vi "Auto Setup.vi"(4 "Sequence Context":T2) -> (0 "error out":errorcluster, 1 "Test Data":T1={"PASS/FAIL Flag"=TRUE, "Numeric Measurement"=0.0, "String Measurement"="", "Report Text"=""} {"Numeric Measurement" format="%.2f"})   [LabVIEW 2013]
uses:
  <vilib>/addons/TestStand/_TSLegacy.llb/LabVIEW Test - Sequence Context.ctl
  <vilib>/addons/TestStand/_TSLegacy.llb/LabVIEW Test - Test Data.ctl
panel:
  in  "Power Train Control Module":bool
  in  "Engine Control Module":bool=TRUE
  in  "Fuel Injection":bool
  in  "Ignition System":bool=TRUE
  in  "Charging System":bool
  in  "Accept":bool
  in  "Battery Voltage":dbl(knob)=11.72609352032594 scale=0.0..15.0 scale format="%.1f"
  # "Verify sequence algorithm by setting tests to Fail.\nForce test(s) to Fail by clicking the appropriate checkbox."
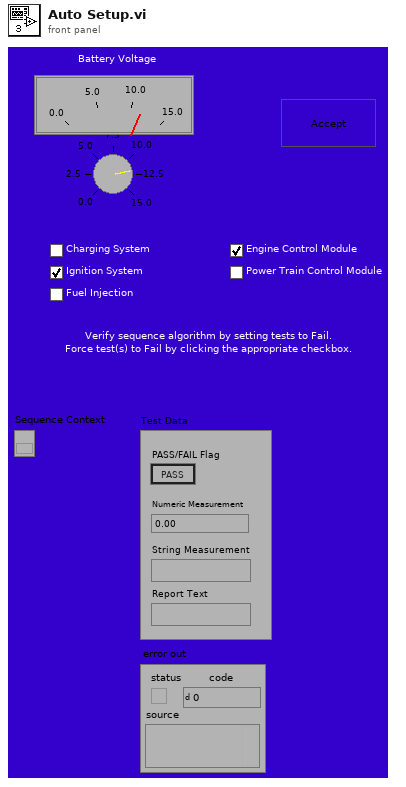
[diagram p1: front panel]
types:
  T1 = typedef "LabVIEW Test - Test Data.ctl" = cluster{"PASS/FAIL Flag":bool, "Numeric Measurement":dbl, "String Measurement":string, "Report Text":string}
  T2 = typedef "LabVIEW Test - Sequence Context.ctl" = refnum<k7>
  T3 = typedef "TestStand - Status Monitor.ctl" = cluster{"Sequence Context":refnum<k7>, "Execution":refnum<k7>, "Termination Monitor":refnum<k7>}
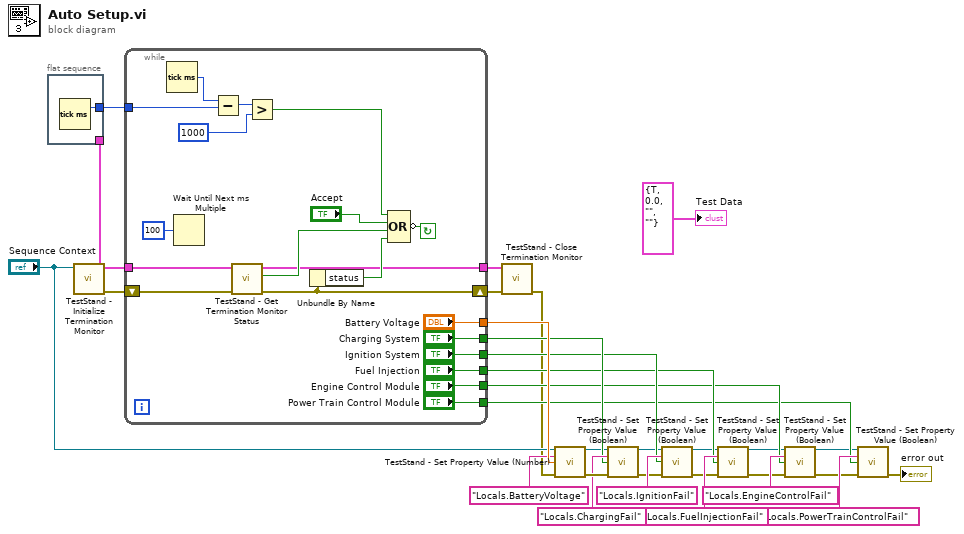
[diagram p0: block diagram]
diagram:
  n1 = flat-sequence {
    tunnel: [w32] -> w1
    tunnel: w2 -> [_]
    frame #0 {
      n2 = Tick Count (ms)() -> (millisecond timer value=w32:u32)
    }
  }
  n3 = call <vilib>:"TestStand - Initialize Termination Monitor.vi"("Sequence Context In"="Sequence Context") -> ("error out"=w7:errorcluster, "Status Monitor Out"=w2:T3)  [unwired: 1 in, 8 out]
  n4 = while {
    tunnel: ["Power Train Control Module"] -> w10
    tunnel: ["Engine Control Module"] -> w12
    tunnel: ["Fuel Injection"] -> w14
    tunnel: ["Ignition System"] -> w16
    tunnel: ["Charging System"] -> w18
    tunnel: ["Battery Voltage"] -> w30
    shift-left: w7 -> [w42]
    shift-right: [w40] -> w5
    tunnel: w2 -> [w41]
    tunnel: [w38] -> w4
    tunnel: w1 -> [w34]
    stop <- w51 continue-if-true
    n5 = Tick Count (ms)() -> (millisecond timer value=w36:u32)
    n6 = Wait Until Next ms Multiple(millisecond multiple=u32 100) -> ()  [unwired: 1 out]
    n7 = Subtract(x=w36, y=w34) -> (x-y=w37:u32)
    n8 = call <vilib>:"TestStand - Get Termination Monitor Status.vi"("error in (no error)"=w42, "Status Monitor In"=w41) -> ("error out"=w40:errorcluster, "Terminating or Aborting"=w39:bool, "Status Monitor Out"=w38:T3)  [unwired: 7 out]
    n9 = Greater?(x=w37, y=u32 1000) -> (0:w33:bool)
    n10 = Unbundle By Name(w40) -> ("status"=w52:bool)
    n11 = Compound Arithmetic op=OR(w33, "Accept", w39, w52) -> (invert w51:bool)
  }
  n12 = call <vilib>:"TestStand - Close Termination Monitor.vi"("error in (no error)"=w5, "Status Monitor In"=w4) -> ("error out"=w3:errorcluster)  [unwired: 9 out]
  n13 = call <vilib>:"TestStand - Set Property Value (Number).vi"("Sequence Context In"="Sequence Context", "Lookup String"="Locals.BatteryVoltage", "New Value"=w30, "error in (no error)"=w3) -> ("Sequence Context Out"=w17:refnum<k7>, "error out"=w28:errorcluster)  [unwired: 1 in, 9 out]
  n14 = call <vilib>:"TestStand - Set Property Value (Boolean).vi"("Sequence Context In"=w17, "Lookup String"="Locals.ChargingFail", "New Value"=w18, "error in (no error)"=w28) -> ("Sequence Context Out"=w15:refnum<k7>, "error out"=w22:errorcluster)  [unwired: 1 in, 9 out]
  n15 = call <vilib>:"TestStand - Set Property Value (Boolean).vi"("Sequence Context In"=w15, "Lookup String"="Locals.IgnitionFail", "New Value"=w16, "error in (no error)"=w22) -> ("Sequence Context Out"=w13:refnum<k7>, "error out"=w21:errorcluster)  [unwired: 1 in, 9 out]
  n16 = call <vilib>:"TestStand - Set Property Value (Boolean).vi"("Sequence Context In"=w13, "Lookup String"="Locals.FuelInjectionFail", "New Value"=w14, "error in (no error)"=w21) -> ("Sequence Context Out"=w11:refnum<k7>, "error out"=w20:errorcluster)  [unwired: 1 in, 9 out]
  n17 = call <vilib>:"TestStand - Set Property Value (Boolean).vi"("Sequence Context In"=w11, "Lookup String"="Locals.EngineControlFail", "New Value"=w12, "error in (no error)"=w20) -> ("Sequence Context Out"=w9:refnum<k7>, "error out"=w19:errorcluster)  [unwired: 1 in, 9 out]
  n18 = call <vilib>:"TestStand - Set Property Value (Boolean).vi"("Sequence Context In"=w9, "Lookup String"="Locals.PowerTrainControlFail", "New Value"=w10, "error in (no error)"=w19) -> ("error out"=→"error out":errorcluster)  [unwired: 1 in, 10 out]
  "Test Data" <- T1 {"PASS/FAIL Flag"=TRUE, "Numeric Measurement"=0.0, "String Measurement"="", "Report Text"=""} ("Test Data")
